vi "Paint Bounding Box.vi"(9 "Camera Image":T3) -> (0 "Thresholded Image":T3(plugin-control), 1 "Bounding Box Final":T4, 2 "Particle Report 2":T1, 3 "Particle Report":T1, 4 "General Report":T2(array[cluster]))   [LabVIEW 2017]
uses:
  <vilib>/vision/Image Controls.llb/IMAQ Image.ctl
panel:
  in  "R/G/B":cluster{"Lower value":i32, "Upper value":i32}[](array[cluster])=[{"Lower value"=0, "Upper value"=40}, {"Lower value"=80, "Upper value"=255}, {"Lower value"=0, "Upper value"=255}]
  out "Particle Report":T2(array[cluster]) {"Orientation" format="%.2f"; "Dimensions"."Height" format="%.2f"; "Dimensions"."Width" format="%.2f"; "Center of Mass"."Y" format="%.2f"; "Center of Mass"."X" format="%.2f"; "Bounding Rect"."Bottom" format="%.2f"; "Bounding Rect"."Right" format="%.2f"; "Bounding Rect"."Top" format="%.2f"; "Bounding Rect"."Left" format="%.2f"; "Number of Holes" format="%.2f"; "Area" format="%.2f"}
  in  "sampleimage":string
  out "Base Image":T3(plugin-control)
  # "difference = width*4"
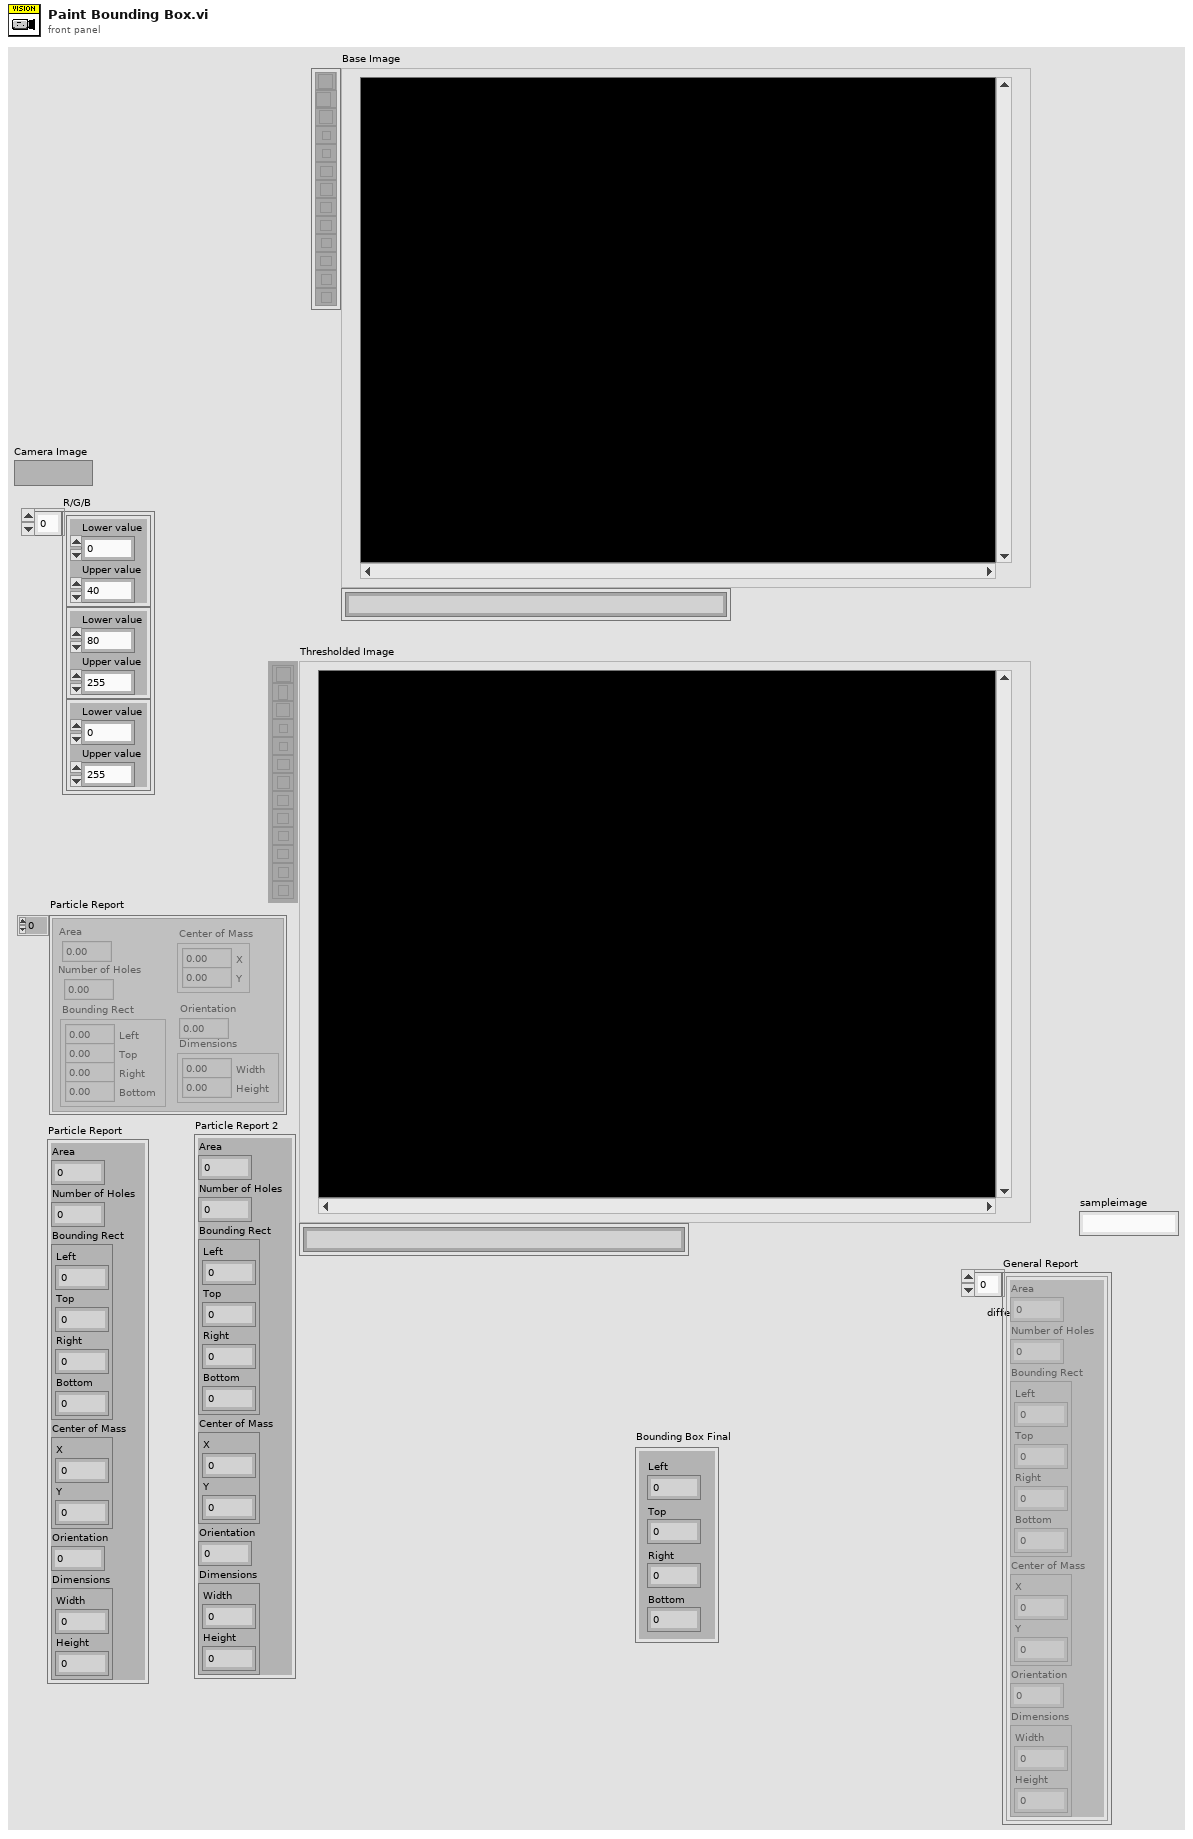
[diagram p1: front panel]
types:
  T1 = cluster{"Area":dbl, "Number of Holes":dbl, "Bounding Rect":cluster{"Left":dbl, "Top":dbl, "Right":dbl, "Bottom":dbl}, "Center of Mass":cluster{"X":dbl, "Y":dbl}, "Orientation":dbl, "Dimensions":cluster{"Width":dbl, "Height":dbl}}
  T2 = cluster{"Area":dbl, "Number of Holes":dbl, "Bounding Rect":cluster{"Left":dbl, "Top":dbl, "Right":dbl, "Bottom":dbl}, "Center of Mass":cluster{"X":dbl, "Y":dbl}, "Orientation":dbl, "Dimensions":cluster{"Width":dbl, "Height":dbl}}[]
  T3 = typedef "IMAQ Image.ctl" = refnum<image>
  T4 = cluster{"Left":dbl, "Top":dbl, "Right":dbl, "Bottom":dbl}
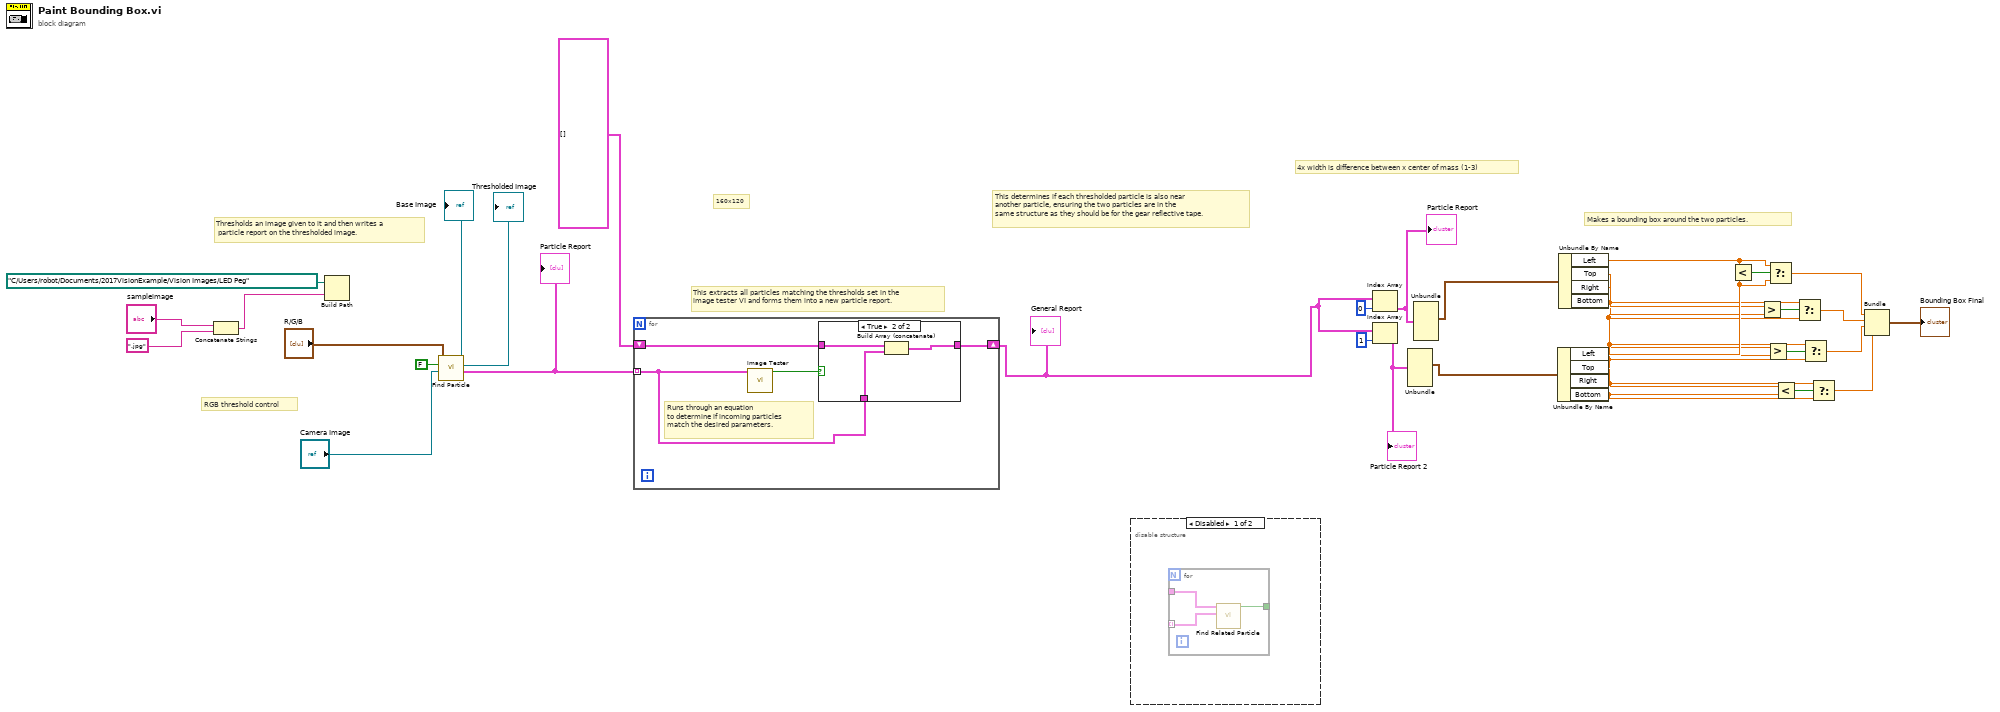
[diagram p0: block diagram]
diagram:
  # "This determines if each thresholded particle is also near \nanother particle, ensuring the two particles are in the \nsame structure as they should be for the gear reflective tape."
  # "Makes a bounding box around the two particles."
  # "4x width is difference between x center of mass (1-3)"
  # "RGB threshold control"
  # "This extracts all particles matching the thresholds set in the \nimage tester VI and forms them into a new particle report."
  # "Thresholds an image given to it and then writes a\n particle report on the thresholded image."
  # "160x120"
  n1 = Concatenate Strings("sampleimage", ".jpg" ("string")) -> (w27:string)
  n2 = Build Path(base path=path "C:/Users/robot/Documents/2017VisionExample/Vision Images/LED Peg", name or relative path=w27) -> ()  [unwired: 1 out]
  n3 = call "Find Particle.vi"("Camera Image"="Camera Image", "From File"=FALSE, "R/G/B"="R/G/B") -> ("Particle Report"=w33:T2, "Thresholded Image"=→"Thresholded Image":T3, "Base Image"=→"Base Image":T3)  [unwired: 4 in, 2 out]
  "Particle Report" <- w33
  n4 = for {
    tunnel: w33 -> [w36] mode=indexing
    shift-right: [w39] -> w1
    shift-left: T2 [] -> [w38]
    # "Runs through an equation\nto determine if incoming particles \nmatch the desired parameters."
    n5 = call "Image Tester.vi"("Particle Report"=w36) -> ("Positive"=w37:bool)  [unwired: 10 in]
    n6 = case shown="True" w37 {
      tunnel: w36 -> [_ w41]
      tunnel: [w40 w43] -> w39
      tunnel: w38 -> [w40 w42]
      frame False {
      }
      frame True {
        n7 = Build Array (concatenate)(w42, w41) -> (w43:T2)
      }
    }
  }
  "General Report" <- w1
  n8 = disable-structure shown="Disabled" {
    frame Disabled {
      n9 = for {
        tunnel: _ -> [w46]
        tunnel: _ -> [w45] mode=indexing
        tunnel: [w44] -> _
        n10 = call "Find Related Particle.vi"("All Reports"=w45, "Base Report"=w46) -> ("Nearby"=w44:bool)  [unwired: 9 in]
      }
    }
    frame Enabled {
    }
  }
  n11 = Index Array(array=w1, index=0) -> (element=w24:T1)
  "Particle Report" <- w24
  n12 = Index Array(array=w1, index=1) -> (element=w23:T1)
  "Particle Report 2" <- w23
  n13 = Unbundle(w23) -> ("Bounding Rect"=w3:T4)  [unwired: 5 out]
  n14 = Unbundle(w24) -> ("Bounding Rect"=w2:T4)  [unwired: 5 out]
  n15 = Unbundle By Name(w3) -> ("Left"=w20:dbl, "Top"=w17:dbl, "Right"=w15:dbl, "Bottom"=w11:dbl)
  n16 = Unbundle By Name(w2) -> ("Left"=w21:dbl, "Top"=w18:dbl, "Right"=w14:dbl, "Bottom"=w12:dbl)
  n17 = Less?(x=w21, y=w20) -> (x < y?=w22:bool)
  n18 = Greater?(x=w18, y=w17) -> (0:w19:bool)
  n19 = Greater?(x=w14, y=w15) -> (0:w16:bool)
  n20 = Select(t=w21, s=w22, f=w20) -> (s? t:f=w10:dbl)
  n21 = Less?(x=w12, y=w11) -> (x < y?=w13:bool)
  n22 = Select(t=w18, s=w19, f=w17) -> (s? t:f=w9:dbl)
  n23 = Select(t=w14, s=w16, f=w15) -> (s? t:f=w8:dbl)
  n24 = Select(t=w12, s=w13, f=w11) -> (s? t:f=w7:dbl)
  n25 = Bundle("Left"=w10, "Top"=w9, "Right"=w8, "Bottom"=w7) -> (→"Bounding Box Final":T4)  [unwired: 1 in]
